vi "Begin.vi"(8 "error in":errorcluster) -> (0 "error out":errorcluster)   [LabVIEW 2019]
doc: "Called before other user functions, this VI is expected to open initial I/O refnums, load in file data, and do all program initialization. Notice that the <B>error out</B> terminal is simply used for data flow. Wiring it to other structures or subVIs ensures that this VI runs first."
uses:
  <vilib>/Rock Robotics/WPI/SafetyOutput/WPI_SafetyOutputConfigMenu.ctl
  Robot Global Data.vi
  <vilib>/Rock Robotics/WPI/DriverStation/WPI_DriverStationRobotMode2.ctl
  <vilib>/Rock Robotics/WPI/Joystick/WPI_JoystickDeviceEnum.ctl
  <vilib>/Rock Robotics/Network Tables/NT Write String Array.vi
  <vilib>/Rock Robotics/SystemInterfaces/DIO/FPGA_DIOPWMChannel.ctl
  <vilib>/Rock Robotics/WPI/RobotDrive/WPI_RobotDriveOpen2MotorWithExistingMotors.vi
  lib/5443_FRC_Labview_lib/Begin/IniSpark.vi
  <vilib>/Rock Robotics/WPI/Switch/WPI_SwitchOpenLimit.vi
  <vilib>/Rock Robotics/SystemInterfaces/DIO/FPGA_DIOChannel.ctl
  <vilib>/Rock Robotics/WPI/Gyro/WPI_GyroAnalogOpen.vi
  <vilib>/Rock Robotics/SystemInterfaces/AI/FPGA_AIGyroChannel.ctl
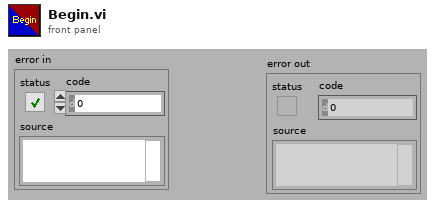
[diagram p1: front panel]
types:
  T1 = typedef "FPGA_AIGyroChannel.ctl" = enum8{"AI 0", "AI 1", "Invalid"}
  T2 = typedef "FPGA_DIOChannel.ctl" = enum8{"DIO 0", "DIO 1", "DIO 2", "DIO 3", "DIO 4", "DIO 5", "DIO 6", "DIO 7", "DIO 8", "DIO 9", "DIO MXP 0", "DIO MXP 1", "DIO MXP 2", "DIO MXP 3", "DIO MXP 4", "DIO MXP 5", "DIO MXP 6", "DIO MXP 7", "DIO MXP 8", "DIO MXP 9", "DIO MXP 10", "DIO MXP 11", "DIO MXP 12", "DIO MXP 13", "DIO MXP 14", "DIO MXP 15", "SPI Port CS1", "SPI Port CS2", "SPI Port CS3", "SPI Port MISO", "SPI Port MOSI", "Invalid"}
  T3 = typedef "FPGA_DIOPWMChannel.ctl" = enum8{"PWM 0", "PWM 1", "PWM 2", "PWM 3", "PWM 4", "PWM 5", "PWM 6", "PWM 7", "PWM 8", "PWM 9", "PWM MXP 0", "PWM MXP 1", "PWM MXP 2", "PWM MXP 3", "PWM MXP 4", "PWM MXP 5", "PWM MXP 6", "PWM MXP 7", "PWM MXP 8", "PWM MXP 9", "Invalid"}
  T4 = typedef "WPI_SafetyOutputConfigMenu.ctl" = enum16{"Enable", "Disable"}
  T5 = typedef "WPI_JoystickDeviceEnum.ctl" = enum16{"USB 0", "USB 1", "USB 2", "USB 3", "USB 4", "USB 5"}
  T6 = typedef "WPI_DriverStationRobotMode2.ctl" = enum16{"Autonomous Disabled", "Autonomous Enabled", "Teleop Disabled", "Teleop Enabled", "Disconnected", "Finish", "Test Disabled", "Test Enabled", "Emergency Stopped"}
  T7 = typedef "WPI_MotorControlDeviceRef.ctl" = cluster{"DeviceStatus":errorcluster, "Type":T8, "PWM":cluster{"PWM Channel":T3, "DeadBand":T9}, "CAN":cluster{"Device Number":u8, "SetOutput VI Ref":variant, "GetOutput VI Ref":variant, "Enable VI Ref":variant, "Disable VI Ref":variant, "Data":variant}, "Invert":bool, "DIO PWM":cluster{"PWM \"Enable\" Channel":T3, "DIOChannel":T2, "PWM Rate":dbl}}
  T8 = typedef "WPI_MotorControlType.ctl" = enum16{"PWM", "CAN", "DIO PWM"}
  T9 = typedef "WPI_PWMDeadband.ctl" = cluster{"Name":string, "maxPositivePwm":i32, "minPositivePwm":i32, "centerPwm":i32, "maxNegativePwm":i32, "minNegativePwm":i32, "angularRange":u16}
  T10 = typedef "WPI_RobotDriveDevRef.ctl" = cluster{"DevStatus":errorcluster, "Motors[]":T7[], "Square Inputs":bool, "Max Output":dbl}
  T11 = typedef "WPI_SwitchDevRef.ctl" = cluster{"DevStatus":errorcluster, "DIO Channel":T2, "CntIndex":T12, "Normally Closed":bool}
  T12 = typedef "FPGA_CounterCtrSystemIndex.ctl" = enum8{"Ctr 0", "Ctr 1", "Ctr 2", "Ctr 3", "Ctr 4", "Ctr 5", "Ctr 6", "Ctr 7", "Invalid"}
  T13 = typedef "WPI_JoystickDevRef.ctl" = cluster{"Device":T5}
  T14 = typedef "WPI_GyroDevRef.ctl" = cluster{"DevStatus":errorcluster, "Analog Channel":T15, "Gain (VoltsPerDegree/Second)":dbl, "Gyro Type":enum16{"Analog", "XRS450"}, "Handle":i32, "SPI Bus":T16, "Device Found":bool, "Sample Rate":dbl, "Calibrate On Open":bool, "Offset":dbl}
  T15 = typedef "FPGA_AIChannel.ctl" = enum8{"AI 0", "AI 1", "AI 2", "AI 3", "AI MXP 0", "AI MXP 1", "AI MXP 2", "AI MXP 3", "Invalid"}
  T16 = typedef "spi_bus.ctl" = enum16{"SPI On-Board, CS0", "SPI On-Board, CS1", "SPI On-Board, CS2", "SPI On-Board, CS3", "SPI MXP", "Invalid"}
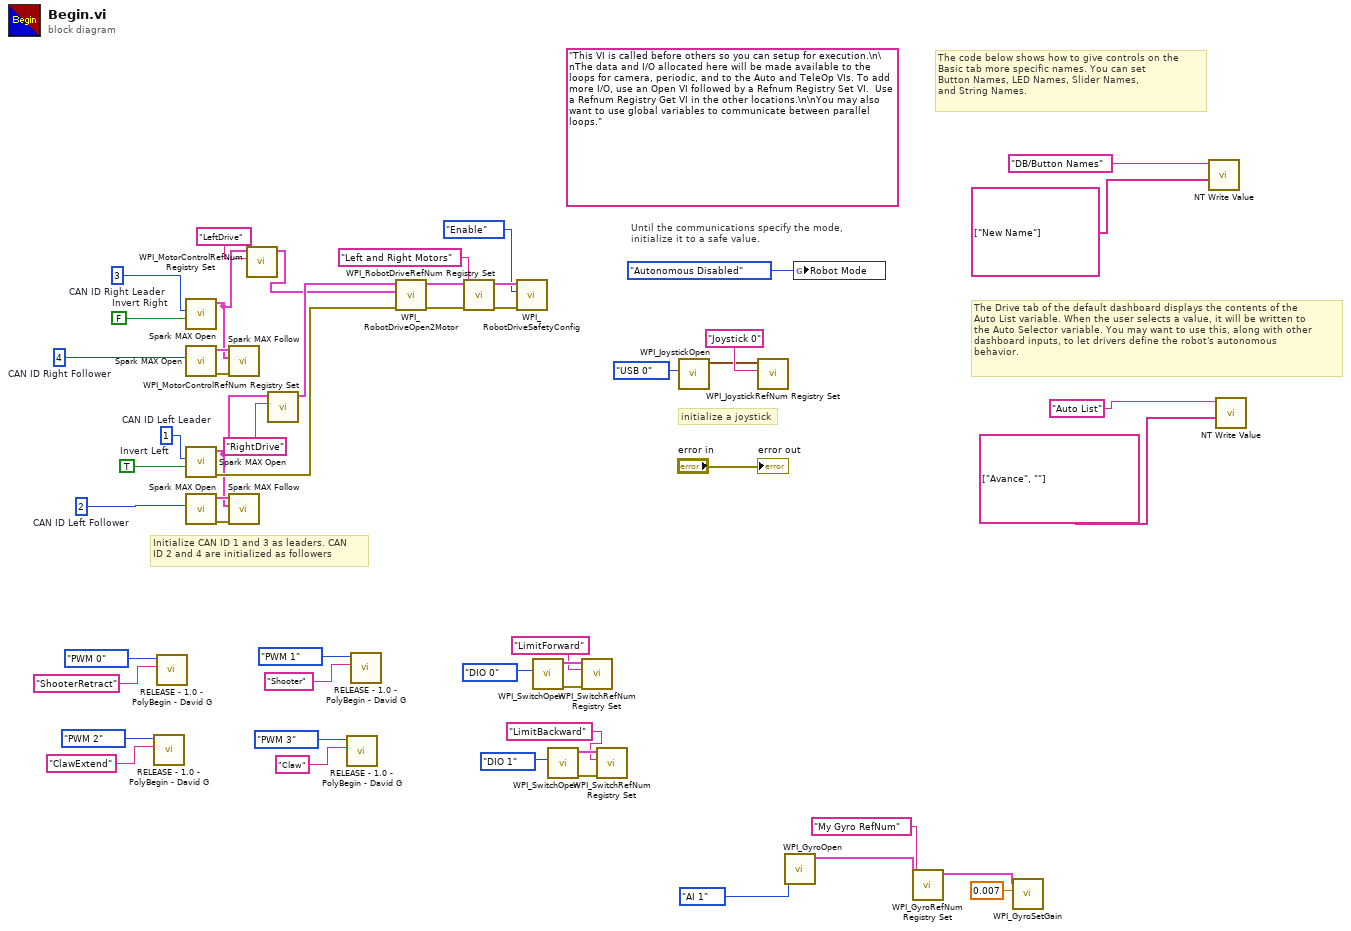
[diagram p0: block diagram]
diagram:
  w28 = TRUE  # Invert Left
  w34 = FALSE  # Invert Right
  w35 = u8 3  # CAN ID Right Leader
  w38 = u8 4  # CAN ID Right Follower
  w29 = u8 1  # CAN ID Left Leader
  w31 = u8 2  # CAN ID Left Follower
  (unwired) "This VI is called before others so you can setup for execution.\n\nThe data and I/O allocated here will be made available to the loops for camera, periodic, and to the Auto and TeleOp VIs. To add more I/O, use an Open VI followed by a Refnum Registry Set VI.  Use a Refnum Registry Get VI in the other locations.\n\nYou may also want to use global variables to communicate between parallel loops."
  # "Initialize CAN ID 1 and 3 as leaders. CAN \nID 2 and 4 are initialized as followers"
  # "The Drive tab of the default dashboard displays the contents of the\nAuto List variable. When the user selects a value, it will be written to\nthe Auto Selector variable. You may want to use this, along with other\ndashboard inputs, to let drivers define the robot's autonomous\nbehavior."
  # "The code below shows how to give controls on the\nBasic tab more specific names. You can set\nButton Names, LED Names, Slider Names,\nand String Names."
  # "initialize a joystick"
  # "Until the communications specify the mode,\ninitialize it to a safe value."
  n1 = call-poly "RELEASE - 1.0 - PolyBegin - David G.vi"("refnum name"="ClawExtend", "PWM Channel"=FPGA_DIOPWMChannel."PWM 2") -> ()  [unwired: 10 in]
  n2 = call-poly "RELEASE - 1.0 - PolyBegin - David G.vi"("refnum name"="ShooterRetract", "PWM Channel"=FPGA_DIOPWMChannel."PWM 0") -> ()  [unwired: 10 in]
  n3 = call "Spark MAX Open.vi"("Invert"=w34, "Device Number"=w35) -> ("MotorControlDeviceRef"=w23:T7)  [unwired: 8 in, 1 out]
  n4 = call "Spark MAX Open.vi"("Device Number"=w38) -> ("error out"=w36:errorcluster, "MotorControlDeviceRef"=w37:T7)  [unwired: 9 in]
  n5 = call "Spark MAX Open.vi"("Invert"=w28, "Device Number"=w29) -> ("error out"=w30:errorcluster, "MotorControlDeviceRef"=w25:T7)  [unwired: 8 in]
  n6 = call "Spark MAX Open.vi"("Device Number"=w31) -> ("error out"=w32:errorcluster, "MotorControlDeviceRef"=w33:T7)  [unwired: 9 in]
  n7 = call "Spark MAX Follow.vi"("error in (no error)"=w36, "Master Controller"=w23, "MotorControlDeviceRef"=w37) -> ()  [unwired: 7 in, 2 out]
  n8 = call "Spark MAX Follow.vi"("error in (no error)"=w32, "Master Controller"=w25, "MotorControlDeviceRef"=w33) -> ()  [unwired: 7 in, 2 out]
  n9 = call <vilib>:"WPI_MotorControlRefNum Registry Set.vi"("refnum name"="LeftDrive", "MotorControlDevRef"=w23) -> ("MotorControlDevRef"=w22:T7)  [unwired: 8 in, 1 out]
  n10 = call <vilib>:"WPI_MotorControlRefNum Registry Set.vi"("refnum name"="RightDrive", "MotorControlDevRef"=w25) -> ("MotorControlDevRef"=w24:T7)  [unwired: 8 in, 1 out]
  n11 = call-poly "RELEASE - 1.0 - PolyBegin - David G.vi"("refnum name"="Claw", "PWM Channel"=FPGA_DIOPWMChannel."PWM 3") -> ()  [unwired: 10 in]
  n12 = call-poly "RELEASE - 1.0 - PolyBegin - David G.vi"("refnum name"="Shooter", "PWM Channel"=FPGA_DIOPWMChannel."PWM 1") -> ()  [unwired: 10 in]
  n13 = call-poly <vilib>:"WPI_RobotDriveOpen2Motor.vi"("error in (no error)"=w30, "Right Motor Dev Ref"=w22, "Left Motor Dev Ref"=w24) -> ("error out"=w41:errorcluster, "RobotDriveDevRef"=w39:T10)  [unwired: 7 in]
  n14 = call <vilib>:"WPI_RobotDriveRefNum Registry Set.vi"("error in (no error)"=w41, "refnum name"="Left and Right Motors", "RobotDriveDevRef"=w39) -> ("error out"=w44:errorcluster, "RobotDriveDevRef"=w43:T10)  [unwired: 7 in]
  n15 = call <vilib>:"WPI_RobotDriveSafetyConfig.vi"("error in (no error)"=w44, "mode"=WPI_SafetyOutputConfigMenu."Enable", "RobotDriveDevRef"=w43) -> ()  [unwired: 7 in, 2 out]
  n16 = call-poly <vilib>:"WPI_SwitchOpen.vi"("DIO Channel"=FPGA_DIOChannel."DIO 0") -> ("error out"=w11:errorcluster, "SwitchDevRef"=w10:T11)  [unwired: 9 in]
  n17 = call-poly <vilib>:"WPI_SwitchOpen.vi"("DIO Channel"=FPGA_DIOChannel."DIO 1") -> ("error out"=w13:errorcluster, "SwitchDevRef"=w12:T11)  [unwired: 9 in]
  n18 = call <vilib>:"WPI_SwitchRefNum Registry Set.vi"("error in (no error)"=w11, "refnum name"="LimitForward", "SwitchDevRef"=w10) -> ()  [unwired: 7 in, 2 out]
  n19 = call <vilib>:"WPI_SwitchRefNum Registry Set.vi"("error in (no error)"=w13, "refnum name"="LimitBackward", "SwitchDevRef"=w12) -> ()  [unwired: 7 in, 2 out]
  n20 = call <vilib>:"WPI_JoystickOpen.vi"("JoystickDevice"=WPI_JoystickDeviceEnum."USB 0") -> ("JoystickDevRef"=w51:T13)  [unwired: 10 in]
  n21 = call <vilib>:"WPI_JoystickRefNum Registry Set.vi"("refnum name"="Joystick 0", "JoystickDevRef"=w51) -> ()  [unwired: 8 in, 2 out]
  n22 = call-poly <vilib>:"WPI_GyroOpen.vi"("Analog Channel"=FPGA_AIGyroChannel."AI 1") -> ("GyroDevRef"=w4:T14)  [unwired: 8 in, 2 out]
  n23 = global write "Robot Global Data.vi" "Robot Mode"(WPI_DriverStationRobotMode2."Autonomous Disabled" ("Robot Mode")) -> ()
  n24 = call <vilib>:"WPI_GyroRefNum Registry Set.vi"("refnum name"="My Gyro RefNum", "GyroDevRef"=w4) -> ("GyroDevRef"=w3:T14)  [unwired: 8 in, 1 out]
  n25 = call <vilib>:"WPI_GyroSetGain.vi"("Gain (VoltsPerDegree/Second)"=0.007, "GyroDevRef"=w3) -> ()  [unwired: 8 in, 2 out]
  n26 = call-poly <vilib>:"NT Write Value.vi"("String Array"=string[] ["New Name"], "Name"="DB/Button Names") -> ()  [unwired: 9 in, 1 out]
  n27 = call-poly <vilib>:"NT Write Value.vi"("String Array"=string[] ["Avance", ""], "Name"="Auto List") -> ()  [unwired: 9 in, 1 out]
  "error out" <- "error in"
